vi "Write Forward Drive State.vi"(8 "error in (no error)":errorcluster, 10 "Forward Drive State":T1 {"Right Drive Power" min=-1.0 max=1.0 scale=-1.0..1.0; "Left Drive Power" min=-1.0 max=1.0 scale=-1.0..1.0}, 11 "Forward Drive in":refnum<class "Forward Drive.lvclass">) -> (0 "error out":errorcluster, 3 "Forward Drive out":refnum<class "Forward Drive.lvclass">)   [LabVIEW 2014, in "Forward Drive.lvlib" / "Forward Drive.lvclass"]
uses:
  Forward Drive.lvclass
  Virtual Robot/Virtual Forward Drive/Virtual Forward Drive Class/Forward Drive State.ctl
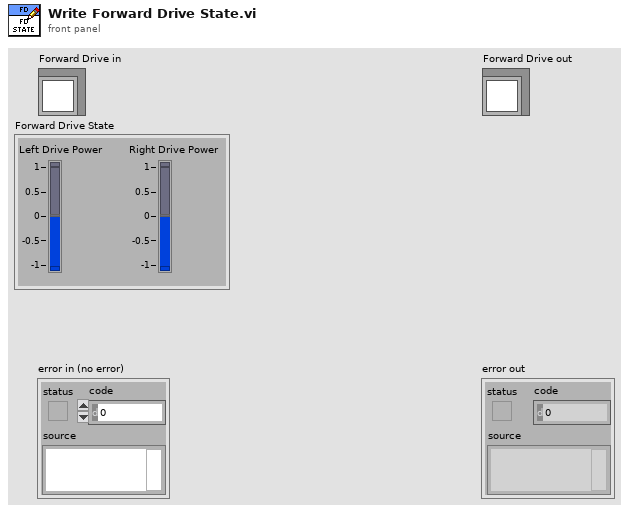
[diagram p1: front panel]
types:
  T1 = typedef "Forward Drive.lvlib/Forward Drive.lvclass/Forward Drive State.ctl" = cluster{"Left Drive Power":dbl, "Right Drive Power ":dbl}
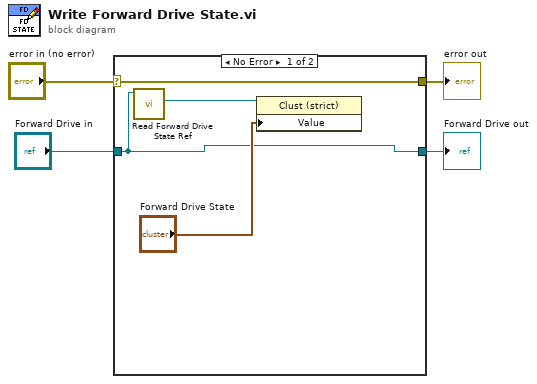
[diagram p0: block diagram]
diagram:
  n1 = case shown="No Error" "error in (no error)" {
    selector: "error in (no error)" -> [w8 w10]
    tunnel: [w8 w10] -> w3
    tunnel: [w5 w9] -> w1
    tunnel: "Forward Drive in" -> [w5 w9]
    frame No Error {
      n2 = call-dynamic "Read Forward Drive State Ref.vi"("Logical Forward Drive in"=w5) -> ("Forward Drive State Ref"=w7:refnum<vi>)  [unwired: 8 in, 2 out]
      n3 = property class="Clust (strict)"(reference=w7, "Value"="Forward Drive State") -> ()  [unwired: 1 in, 2 out]
    }
    frame Error {
    }
  }
  "error out" <- w3
  "Forward Drive out" <- w1
